vi "GOMDBTS2048 set Trigger Internal Levels.vi"(8 "error in (no error)":errorcluster, 9 "lightValueMax":dbl, 10 "lightValueTrigger":dbl, 11 "handle":i32) -> (0 "error out":errorcluster, 3 "function return":i32)   [LabVIEW 2015, in "GOMDBTS2048.lvlib"]
doc: "GOBTS2048DLL int __stdcall GOMDBTS2048_setTriggerInternalLevels(int handle, int lightValueTrigger, int lightValueMax);"
uses:
  GOMDBTS2048.lvlib
  runtime/GOMDBTS2048.dll
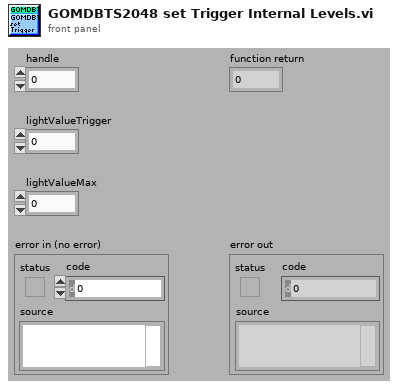
[diagram p1: front panel]
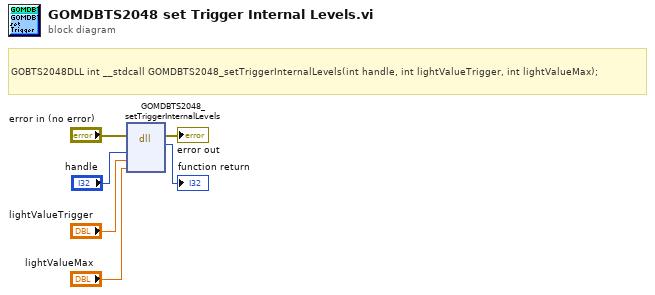
[diagram p0: block diagram]
diagram:
  # "GOBTS2048DLL int __stdcall GOMDBTS2048_setTriggerInternalLevels(int handle, int lightValueTrigger, int lightValueMax);"
  n1 = dll-call lib="C:/Users/rkoch/Documents/GO_Library/runtime/GOMDBTS2048.*" fn="GOMDBTS2048_setTriggerInternalLevels"(error in="error in (no error)", "handle"="handle", "lightValueTrigger"="lightValueTrigger", "lightValueMax"="lightValueMax") -> (error out=→"error out":errorcluster, "return type"=→"function return":i32)  [unwired: 5 in, 1 out]
